vi "Set IO Enable.vi"(6 "Write to FPGA(T)":bool=TRUE, 8 "error in (no error)":errorcluster, 10 "Write Enable":u32, 11 "FPGA VI Reference In":refnum<k20>) -> (0 "error out":errorcluster, 3 "FPGA VI Reference Out":refnum<k20>)   [LabVIEW 2016]
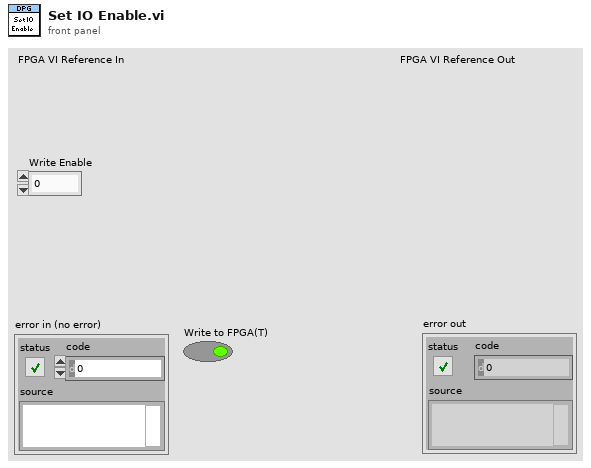
[diagram p1: front panel]
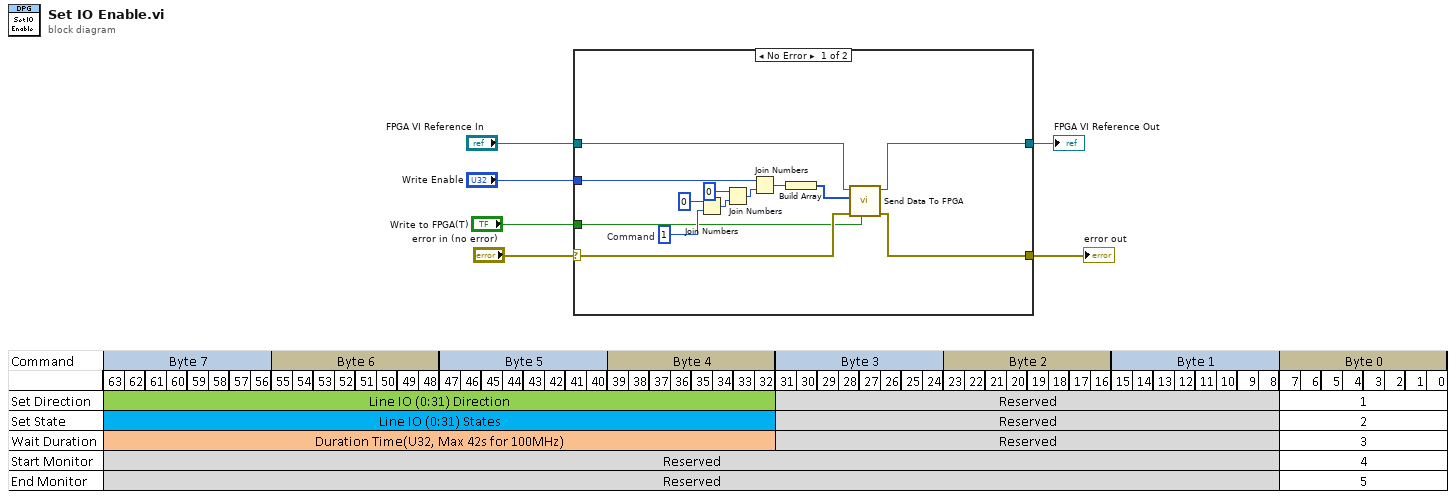
[diagram p0: block diagram]
diagram:
  n1 = case shown="No Error" "error in (no error)" {
    selector: "error in (no error)" -> [w10 w21]
    tunnel: "FPGA VI Reference In" -> [w13 w20]
    tunnel: [w8 w21] -> w4
    tunnel: "Write Enable" -> [w19 _]
    tunnel: "Write to FPGA(T)" -> [w9 _]
    tunnel: [w7 w20] -> w1
    frame No Error {
      w16 = u16 1  # Command
      n2 = Join Numbers(hi=u16 0, lo=w16) -> ((hi.lo)=w17:u32)
      n3 = Join Numbers(hi=u32 0, lo=w17) -> ((hi.lo)=w18:u64)
      n4 = Join Numbers(hi=w19, lo=w18) -> ((hi.lo)=w12:u64)
      n5 = Build Array(w12) -> (w11:u64[])
      n6 = call "Send Data To FPGA.vi"("Write to FPGA(T)"=w9, "error in (no error)"=w10, "Data"=w11, "FPGA VI Reference In"=w13) -> ("error out"=w8:errorcluster, "FPGA VI Reference Out"=w7:refnum<k20>)  [unwired: 6 in]
    }
    frame Error {
    }
  }
  "error out" <- w4
  "FPGA VI Reference Out" <- w1
